vi "2photocell+ledcontrol.vi"() -> ()   [LabVIEW 2016]
uses:
  <vilib>/LabVIEW Interface for Arduino/LabVIEW Interface for Arduino.lvlib
  <vilib>/ptbypt/NI_PtbyPt.lvlib
panel:
  in  "Tab Control":enum32{"Page 1", "Page 2"}(tab)
  out "Voltage":dbl(knob) scale=0.0..5.0
  out "Filtered x":dbl format="%0.2f"
  out "Voltage 2":dbl(knob) scale=0.0..5.0
  out "Filtered x 2":dbl format="%0.2f"
  in  "thrs low":i32=1
  in  "thrs high":i32=4
  in  "stop":bool
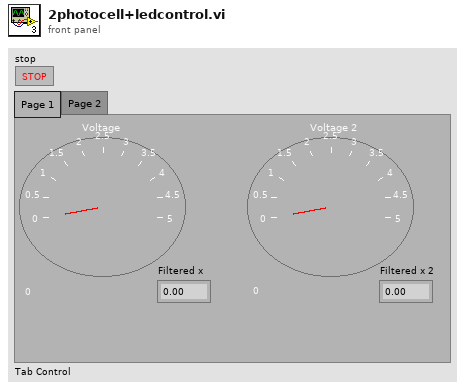
[diagram p1: front panel]
types:
  T1 = typedef "LabVIEW Interface for Arduino.lvlib/Arduino Resource.ctl" = cluster{"VISA resource":refnum<visa-resource-name>, "Board Type":T2, "Connection Type":enum8{"USB / Serial"}, "Bytes Per Packet (15)":u8}
  T2 = typedef "LabVIEW Interface for Arduino.lvlib/Board Type.ctl" = enum16{"Uno", "Dimuelanove w/Atmega 328", "Mega 2560"}
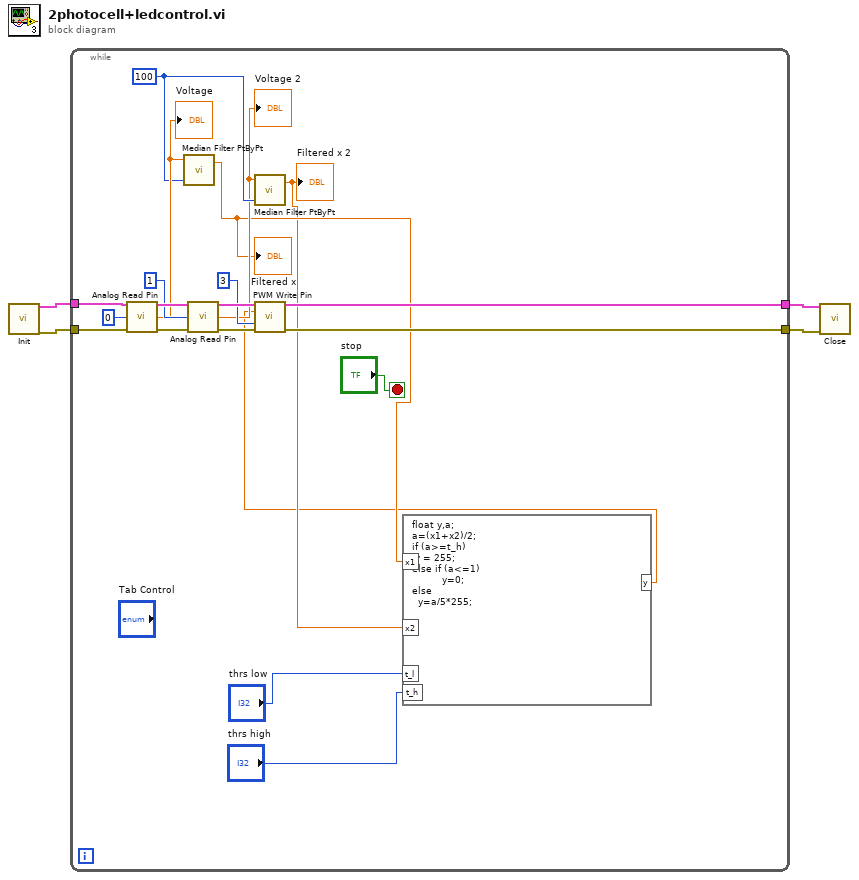
[diagram p0: block diagram]
diagram:
  n1 = call <vilib>:"Init.vi"() -> ("Arduino Resource"=w3:T1, "error out"=w4:errorcluster)  [unwired: 18 in]
  n2 = while {
    tunnel: w4 -> [w20]
    tunnel: w3 -> [w15]
    tunnel: [w12] -> w2
    tunnel: [w11] -> w1
    stop <- "stop" stop-if-true
    w13 = 100 ("rank")
    n3 = call <vilib>:"Analog Read Pin.vi"("Arduino Resource"=w15, "Analog Input Pin (0)"=u8 0, "error in"=w20) -> ("Arduino Resource"=w24:T1, "Voltage"=w14:dbl, "error out"=w19:errorcluster)  [unwired: 10 in]
    "Voltage" <- w14
    n4 = call <vilib>:"Median Filter PtByPt.vi"("rank"=w13, "x"=w14) -> ("Filtered x"=w9:dbl)  [unwired: 2 in, 1 out]
    "Filtered x" <- w9
    n5 = call <vilib>:"Analog Read Pin.vi"("Arduino Resource"=w24, "Analog Input Pin (0)"=u8 1, "error in"=w19) -> ("Arduino Resource"=w18:T1, "Voltage"=w10:dbl, "error out"=w17:errorcluster)  [unwired: 10 in]
    "Voltage 2" <- w10
    n6 = call <vilib>:"Median Filter PtByPt.vi"("rank"=w13, "x"=w10) -> ("Filtered x"=w8:dbl)  [unwired: 2 in, 1 out]
    "Filtered x 2" <- w8
    n7 = formula code="float y,a;\na=(x1+x2)/2;\nif (a>=t_h)\n y = 255;\nelse if (a<=1)\n          y=0;\nelse\n  y=a/5*255;"("x1"=w9, "x2"=w8, "t_l"="thrs low", "t_h"="thrs high") -> ("y"=w7:dbl)
    n8 = call <vilib>:"PWM Write Pin.vi"("Arduino Resource"=w18, "Duty Cycle (0 - 255)"=w7, "PWM Pin (3)"=u8 3, "error in"=w17) -> ("Arduino Resource"=w12:T1, "error out"=w11:errorcluster)  [unwired: 10 in]
  }
  n9 = call <vilib>:"Close.vi"("Arduino Resource"=w2, "error in"=w1) -> ()  [unwired: 13 in, 1 out]
